vi "Start Async.vi"(8 "error in (no error)":errorcluster, 11 "gRPC Server in":refnum<class "OCV4.lvclass">) -> (0 "error out":errorcluster, 3 "gRPC Server out":refnum<class "OCV4.lvclass">)   [LabVIEW 2019, in "OCV4.lvlib" / "OCV4.lvclass"]
uses:
  OCV4.lvclass
  <vilib>/NI_Real-Time Target Support.lvlib
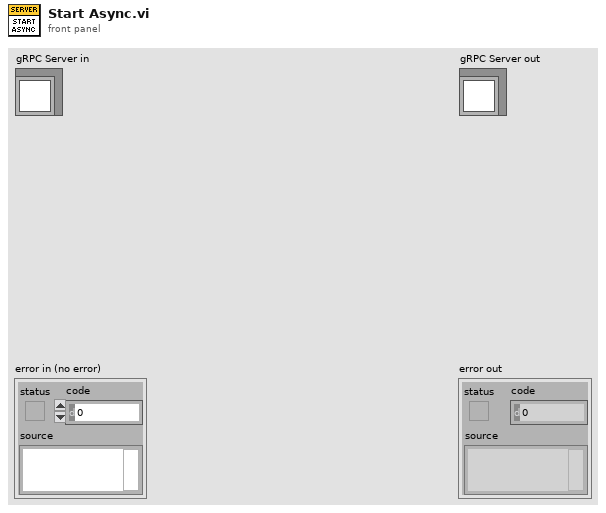
[diagram p1: front panel]
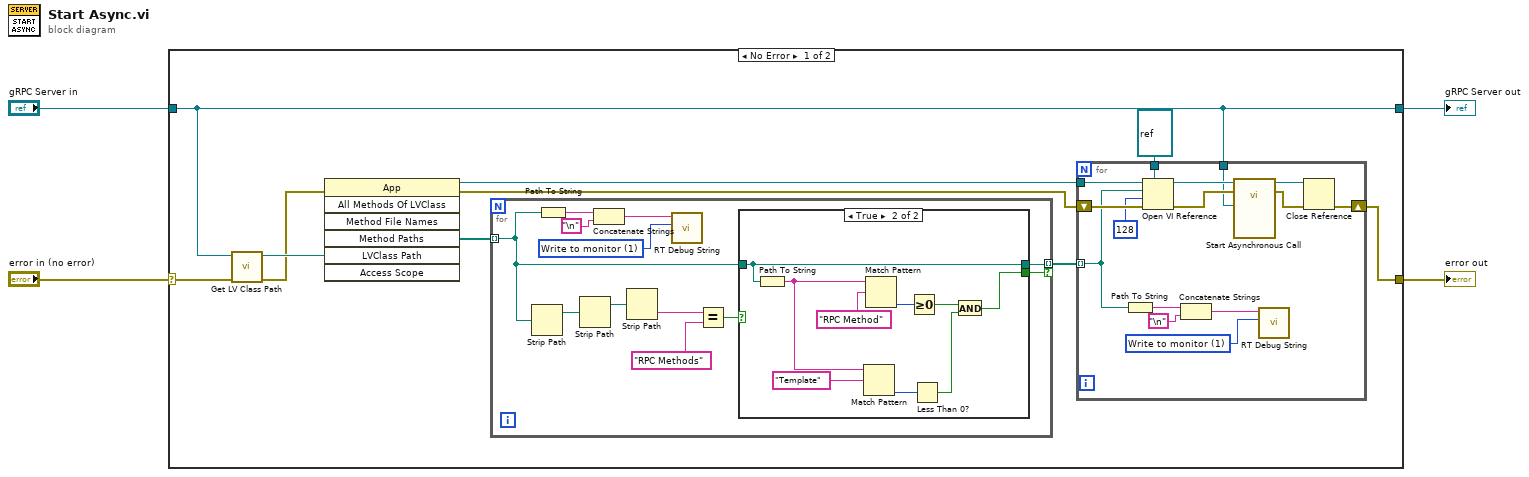
[diagram p0: block diagram]
diagram:
  n1 = case shown="No Error" "error in (no error)" {
    selector: "error in (no error)" -> [w10 w53]
    tunnel: [w7 w53] -> w3
    tunnel: [w11 w52] -> w1
    tunnel: "gRPC Server in" -> [w11 w52]
    frame No Error {
      n2 = call <vilib>:"Get LV Class Path.vi"("error in (no error)"=w10, "object"=w11) -> ("error out"=w8:errorcluster, "class path"=w14:path)  [unwired: 8 in]
      n3 = invoke class="App" method="All Methods Of LVClass"(error in=w8, "LVClass Path"=w14) -> (reference out=w12:refnum<vi>, error out=w9:errorcluster, "Method Paths"=w6:path[])  [unwired: 5 in, 4 out]
      n4 = for {
        tunnel: w6 -> [w15] mode=indexing
        tunnel: [w20] -> w5 mode=indexing if=w26
        w17 = u16 1 items=["Write to serial", "Write to monitor", "Write to system log"] ("Interface")
        n5 = Strip Path(path=w15) -> (stripped path=w25:path)  [unwired: 1 out]
        n6 = Path To String(path=w15) -> (string=w18:string)
        n7 = Strip Path(path=w25) -> (stripped path=w24:path)  [unwired: 1 out]
        n8 = Concatenate Strings(w18, "\n") -> (w19:string)
        n9 = Strip Path(path=w24) -> (name=w22:string)  [unwired: 1 out]
        n10 = call <vilib>:"RT Debug String.vi"("Interface"=w17, "String to write"=w19) -> ()  [unwired: 9 in, 1 out]
        n11 = Equal?(x=w22, y="RPC Methods" ("name")) -> (x = y?=w21:bool)
        n12 = case shown="True" w21 {
          tunnel: [_ w28] -> w26
          tunnel: w15 -> [w27 w34]
          tunnel: [w27 w34] -> w20
          frame False {
          }
          frame True {
            n13 = Path To String(path=w34) -> (string=w33:string)
            n14 = Match Pattern(string=w33, regular expression="Template") -> (offset past match=w31:i32)  [unwired: 1 in, 3 out]
            n15 = Match Pattern(string=w33, regular expression="RPC Method") -> (offset past match=w35:i32)  [unwired: 1 in, 3 out]
            n16 = Greater Or Equal To 0?(x=w35) -> (x >= 0?=w30:bool)
            n17 = Less Than 0?(x=w31) -> (x < 0?=w29:bool)
            n18 = And(x=w30, y=w29) -> (x .and. y?=w28:bool)
          }
        }
      }
      n19 = for {
        tunnel: w5 -> [w38] mode=indexing
        tunnel: refnum<vi> refnum ("type specifier VI Refnum (for type only)") -> [w51]
        tunnel: w12 -> [w48]
        tunnel: w11 -> [w45]
        shift-right: [w43] -> w7
        shift-left: w9 -> [w44]
        w37 = u16 1 items=["Write to serial", "Write to monitor", "Write to system log"] ("Interface")
        n20 = Path To String(path=w38) -> (string=w40:string)
        n21 = Open VI Reference(type specifier VI Refnum (for type only)=w51, application reference (local)=w48, vi path=w38, options=128 ("call and forget"), error in (no error)=w44) -> (vi reference=w50:refnum<vi>, error out=w47:errorcluster)  [unwired: 1 in]
        n22 = Concatenate Strings(w40, "\n") -> (w39:string)
        n23 = call-by-ref "Start Asynchronous Call"(reference=w50, error in=w47, "OOP Server in"=w45) -> (reference out=w49:refnum<vi>, error out=w46:errorcluster)  [unwired: 9 in, 2 out]
        n24 = call <vilib>:"RT Debug String.vi"("Interface"=w37, "String to write"=w39) -> ()  [unwired: 9 in, 1 out]
        n25 = Close Reference(reference=w49, error in (no error)=w46) -> (error out=w43:errorcluster)
      }
    }
    frame Error {
    }
  }
  "error out" <- w3
  "gRPC Server out" <- w1
